vi "Update.vi"(8 "error in (no error)":errorcluster, 10 "Message in":refnum<class "UpdateMessage.lvclass">, 11 "Autofocus in":refnum<class "Autofocus.lvclass">) -> (0 "error out":errorcluster, 3 "Autofocus out":refnum<class "Autofocus.lvclass">)   [LabVIEW 2012, in "Autofocus.lvclass"]
doc: "The update method processes the command 'update'. \n\nThe command 'update' is used for receiving new values to be set to the private data of the class. This could be seen as a public set method for setting new parameters to the private class data."
uses:
  Autofocus.lvclass
  <vilib>/Distrio/Murmex/UpdateMessage/UpdateMessage.lvclass
  Sharpness Measure.ctl
  Autofocus.lvclass/Autofocus.ctl
  image acquisition mode.ctl
  ROI size.ctl
  Search algorithm.ctl
  <vilib>/Distrio/Murmex/Murmex/Murmex.lvclass
panel:
  # "This method is called when the UPDATE\ntrigger is sent. \n\nOverride this method when your component needs to\nrespond to this trigger. \n\nCall parent for proper implementation"
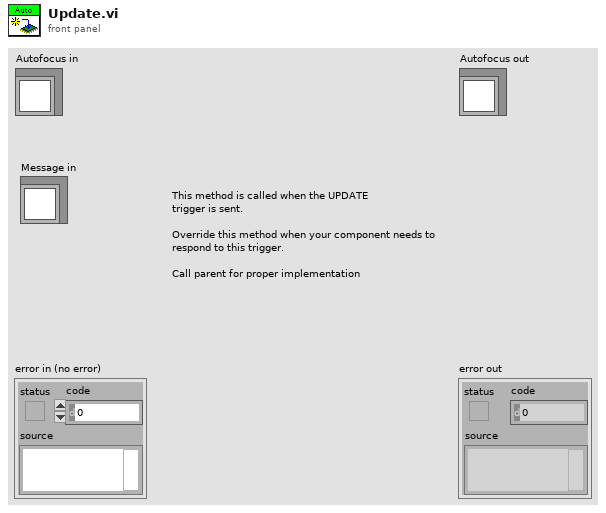
[diagram p1: front panel]
types:
  T1 = typedef "Autofocus.lvclass/Sharpness Measure.ctl" = enum16{"Vol4", "Gradient Square"}
  T2 = typedef "Autofocus.lvclass/image acquisition mode.ctl" = enum16{"Focus Stack", "Single Frame"}
  T3 = typedef "Autofocus.lvclass/Search algorithm.ctl" = enum16{"Hill Climbing", "HC+GS"}
  T4 = typedef "Autofocus.lvclass/ROI size.ctl" = u16
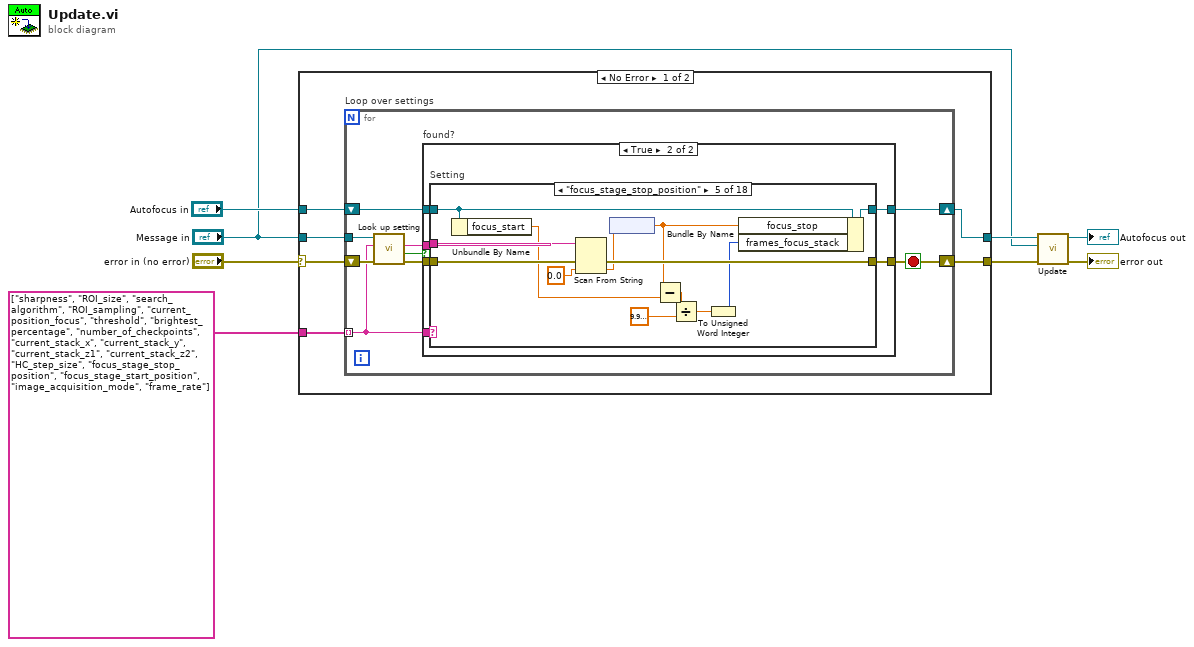
[diagram p0: block diagram]
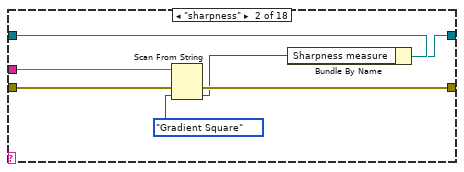
[diagram p4: hidden frame]
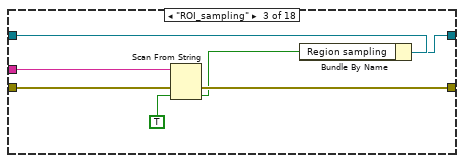
[diagram p5: hidden frame]
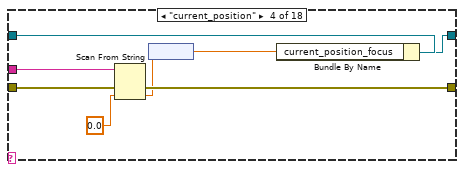
[diagram p6: hidden frame]
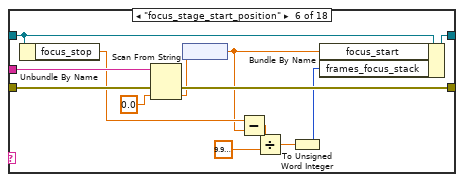
[diagram p7: hidden frame]
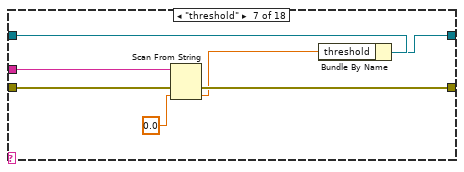
[diagram p8: hidden frame]
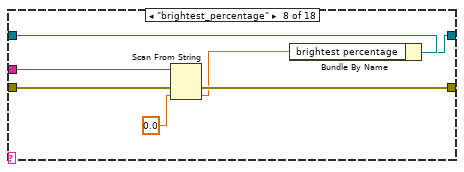
[diagram p9: hidden frame]
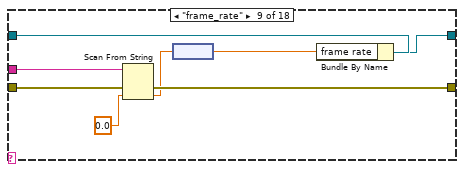
[diagram p10: hidden frame]
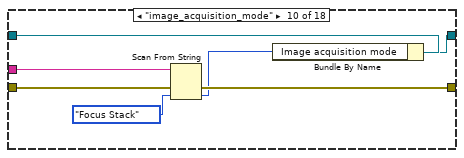
[diagram p11: hidden frame]
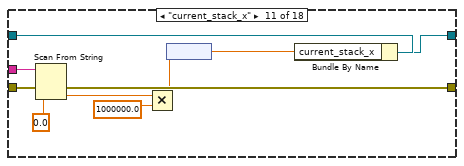
[diagram p12: hidden frame]
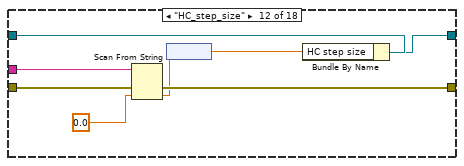
[diagram p13: hidden frame]
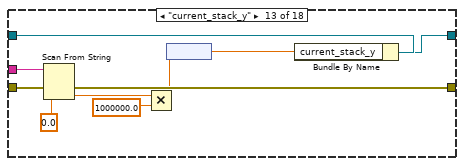
[diagram p14: hidden frame]
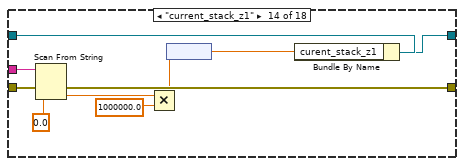
[diagram p15: hidden frame]
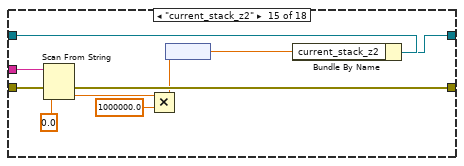
[diagram p16: hidden frame]
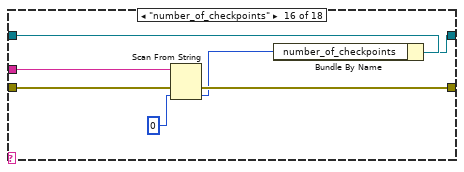
[diagram p17: hidden frame]
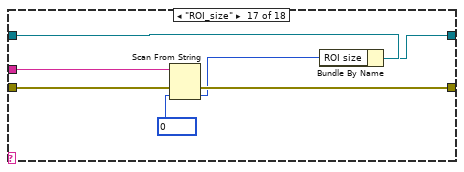
[diagram p18: hidden frame]
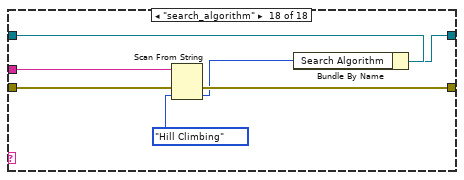
[diagram p19: hidden frame]
diagram:
  n1 = case shown="No Error" "error in (no error)" {
    selector: "error in (no error)" -> [w14 w181]
    tunnel: "Autofocus in" -> [w10 w180]
    tunnel: [w13 w181] -> w5
    tunnel: string[] ["sharpness", "ROI_size", "search_algorithm", "ROI_sampling", "current_position_focus", "threshold", "brightest_percentage", "number_of_checkpoints", "current_stack_x", "current_stack_y", "current_stack_z1", "current_stack_z2", "HC_step_size", "focus_stage_stop_position", "focus_stage_start_position", "image_acquisition_mode", "frame_rate"] -> [w12 _]
    tunnel: "Message in" -> [w11 _]
    tunnel: [w9 w180] -> w3
    frame No Error {
      n2 = for "Loop over settings" {
        shift-right: [w17] -> w13
        shift-left: w14 -> [w23]
        shift-right: [w18] -> w9
        shift-left: w10 -> [w21]
        tunnel: w12 -> [w16] mode=indexing
        tunnel: w11 -> [w15]
        stop <- w17 stop-if-true
        n3 = call <vilib>:"Look up setting.vi"("error in (no error)"=w23, "tag name"=w16, "UpdateMessage in"=w15) -> ("error out"=w19:errorcluster, "found?"=w22:bool, "value"=w20:string)  [unwired: 5 in, 1 out]
        n4 = case "found?" shown="True" w22 {
          tunnel: w21 -> [w25 w29]
          tunnel: w20 -> [_ w30]
          tunnel: w19 -> [w24 w28]
          tunnel: w16 -> [_ w31]
          tunnel: [w25 w27] -> w18
          tunnel: [w24 w26] -> w17
          frame False {
          }
          frame True {
            n5 = case "Setting" shown="\"focus_stage_stop_position\"" w31 {
              tunnel: w30 -> [_ w39 w45 w53 w66 w79 w86 w93 w101 w108 w118 w126 w136 w146 w156 w163 w166 w177]
              tunnel: w29 -> [w33 w38 w43 w52 w57 w76 w85 w92 w100 w107 w117 w125 w135 w145 w155 w162 w169 w175]
              tunnel: w28 -> [w32 w40 w47 w55 w68 w81 w88 w95 w103 w110 w120 w128 w138 w148 w158 w165 w172 w179]
              tunnel: [w33 w37 w42 w51 w65 w78 w84 w91 w99 w106 w116 w124 w134 w144 w154 w161 w167 w174] -> w27
              tunnel: [w32 w36 w46 w54 w67 w80 w87 w94 w102 w109 w119 w127 w137 w147 w157 w164 w171 w178] -> w26
              frame Default {
              }
              frame "sharpness" {
                n6 = Scan From String(input string=w39, error in=w40, default 1=Sharpness_Measure."Gradient Square" ("Sharpness measure")) -> (error out=w36:errorcluster, output 1=w34:T1)  [unwired: 2 in, 2 out]
                n7 = Bundle By Name(cluster=w38, "Sharpness measure"=w34) -> (w37:refnum<class "Autofocus.lvclass">)
              }
              frame "ROI_sampling" {
                n8 = Scan From String(input string=w45, error in=w47, default 1=TRUE) -> (error out=w46:errorcluster, output 1=w41:bool)  [unwired: 2 in, 2 out]
                n9 = Bundle By Name(cluster=w43, "Region sampling"=w41) -> (w42:refnum<class "Autofocus.lvclass">)
              }
              frame "current_position" {
                n10 = Scan From String(input string=w53, error in=w55, default 1=0.0 ("Settings cluster.current_position")) -> (error out=w54:errorcluster, output 1=w49:dbl)  [unwired: 2 in, 2 out]
                n11 = node(w49) -> (w48:dbl[unit])
                n12 = Bundle By Name(cluster=w52, "current_position_focus"=w48) -> (w51:refnum<class "Autofocus.lvclass">)
              }
              frame "focus_stage_stop_position" {
                n13 = Unbundle By Name(w57) -> ("focus_start"=w56:dbl[unit])
                n14 = Scan From String(input string=w66, error in=w68, default 1=0.0 ("Settings cluster.current_position")) -> (error out=w67:errorcluster, output 1=w63:dbl)  [unwired: 2 in, 2 out]
                n15 = node(w63) -> (w58:dbl[unit])
                n16 = Subtract(x=w58, y=w56) -> (x-y=w62:dbl[unit])
                n17 = Divide(x=w62, y=dbl[unit] 9.999999999999999e-06) -> (x/y=w60:dbl)
                n18 = To Unsigned Word Integer(number=w60) -> (unsigned 16bit integer=w59:u16)
                n19 = Bundle By Name(cluster=w57, "focus_stop"=w58, "frames_focus_stack"=w59) -> (w65:refnum<class "Autofocus.lvclass">)
              }
              frame "focus_stage_start_position" {
                n20 = Unbundle By Name(w76) -> ("focus_stop"=w74:dbl[unit])
                n21 = Scan From String(input string=w79, error in=w81, default 1=0.0 ("Settings cluster.current_position")) -> (error out=w80:errorcluster, output 1=w77:dbl)  [unwired: 2 in, 2 out]
                n22 = node(w77) -> (w73:dbl[unit])
                n23 = Subtract(x=w74, y=w73) -> (x-y=w72:dbl[unit])
                n24 = Divide(x=w72, y=dbl[unit] 9.999999999999999e-06) -> (x/y=w70:dbl)
                n25 = To Unsigned Word Integer(number=w70) -> (unsigned 16bit integer=w69:u16)
                n26 = Bundle By Name(cluster=w76, "focus_start"=w73, "frames_focus_stack"=w69) -> (w78:refnum<class "Autofocus.lvclass">)
              }
              frame "threshold" {
                n27 = Scan From String(input string=w86, error in=w88, default 1=0.0 ("Settings cluster.current_position")) -> (error out=w87:errorcluster, output 1=w82:dbl)  [unwired: 2 in, 2 out]
                n28 = Bundle By Name(cluster=w85, "threshold"=w82) -> (w84:refnum<class "Autofocus.lvclass">)
              }
              frame "brightest_percentage" {
                n29 = Scan From String(input string=w93, error in=w95, default 1=0.0 ("Settings cluster.current_position")) -> (error out=w94:errorcluster, output 1=w89:dbl)  [unwired: 2 in, 2 out]
                n30 = Bundle By Name(cluster=w92, "brightest percentage"=w89) -> (w91:refnum<class "Autofocus.lvclass">)
              }
              frame "frame_rate" {
                n31 = Scan From String(input string=w101, error in=w103, default 1=0.0 ("Settings cluster.current_position")) -> (error out=w102:errorcluster, output 1=w97:dbl)  [unwired: 2 in, 2 out]
                n32 = node(w97) -> (w96:dbl[unit])
                n33 = Bundle By Name(cluster=w100, "frame rate"=w96) -> (w99:refnum<class "Autofocus.lvclass">)
              }
              frame "image_acquisition_mode" {
                n34 = Scan From String(input string=w108, error in=w110, default 1=image_acquisition_mode."Focus Stack" ("Settings cluster.Image acquisition mode")) -> (error out=w109:errorcluster, output 1=w105:T2)  [unwired: 2 in, 2 out]
                n35 = Bundle By Name(cluster=w107, "Image acquisition mode"=w105) -> (w106:refnum<class "Autofocus.lvclass">)
              }
              frame "current_stack_x" {
                n36 = Scan From String(input string=w118, error in=w120, default 1=0.0 ("Settings cluster.current_stack_x")) -> (error out=w119:errorcluster, output 1=w112:dbl)  [unwired: 2 in, 2 out]
                n37 = Multiply(x=w112, y=1000000.0) -> (x*y=w111:dbl)
                n38 = node(w111) -> (w114:dbl[unit])
                n39 = Bundle By Name(cluster=w117, "current_stack_x"=w114) -> (w116:refnum<class "Autofocus.lvclass">)
              }
              frame "HC_step_size" {
                n40 = Scan From String(input string=w126, error in=w128, default 1=0.0 ("Settings cluster.current_stack_x")) -> (error out=w127:errorcluster, output 1=w123:dbl)  [unwired: 2 in, 2 out]
                n41 = node(w123) -> (w121:dbl[unit])
                n42 = Bundle By Name(cluster=w125, "HC step size"=w121) -> (w124:refnum<class "Autofocus.lvclass">)
              }
              frame "current_stack_y" {
                n43 = Scan From String(input string=w136, error in=w138, default 1=0.0 ("Settings cluster.current_stack_x")) -> (error out=w137:errorcluster, output 1=w130:dbl)  [unwired: 2 in, 2 out]
                n44 = Multiply(x=w130, y=1000000.0) -> (x*y=w129:dbl)
                n45 = node(w129) -> (w132:dbl[unit])
                n46 = Bundle By Name(cluster=w135, "current_stack_y"=w132) -> (w134:refnum<class "Autofocus.lvclass">)
              }
              frame "current_stack_z1" {
                n47 = Scan From String(input string=w146, error in=w148, default 1=0.0 ("Settings cluster.current_stack_x")) -> (error out=w147:errorcluster, output 1=w140:dbl)  [unwired: 2 in, 2 out]
                n48 = Multiply(x=w140, y=1000000.0) -> (x*y=w139:dbl)
                n49 = node(w139) -> (w142:dbl[unit])
                n50 = Bundle By Name(cluster=w145, "curent_stack_z1"=w142) -> (w144:refnum<class "Autofocus.lvclass">)
              }
              frame "current_stack_z2" {
                n51 = Scan From String(input string=w156, error in=w158, default 1=0.0 ("Settings cluster.current_stack_x")) -> (error out=w157:errorcluster, output 1=w151:dbl)  [unwired: 2 in, 2 out]
                n52 = Multiply(x=w151, y=1000000.0) -> (x*y=w150:dbl)
                n53 = node(w150) -> (w152:dbl[unit])
                n54 = Bundle By Name(cluster=w155, "current_stack_z2"=w152) -> (w154:refnum<class "Autofocus.lvclass">)
              }
              frame "number_of_checkpoints" {
                n55 = Scan From String(input string=w163, error in=w165, default 1=u16 0 ("Settings cluster.current_position")) -> (error out=w164:errorcluster, output 1=w159:u16)  [unwired: 2 in, 2 out]
                n56 = Bundle By Name(cluster=w162, "number_of_checkpoints"=w159) -> (w161:refnum<class "Autofocus.lvclass">)
              }
              frame "ROI_size" {
                w170 = T4 0 items=["50x50"=50, "100x100"=100, "250x250"=250] ("ROI size")
                n57 = Scan From String(input string=w166, error in=w172, default 1=w170) -> (error out=w171:errorcluster, output 1=w168:T4)  [unwired: 2 in, 2 out]
                n58 = Bundle By Name(cluster=w169, "ROI size"=w168) -> (w167:refnum<class "Autofocus.lvclass">)
              }
              frame "search_algorithm" {
                n59 = Scan From String(input string=w177, error in=w179, default 1=Search_algorithm."Hill Climbing" ("Search Algorithm")) -> (error out=w178:errorcluster, output 1=w173:T3)  [unwired: 2 in, 2 out]
                n60 = Bundle By Name(cluster=w175, "Search Algorithm"=w173) -> (w174:refnum<class "Autofocus.lvclass">)
              }
            }
          }
        }
      }
    }
    frame Error {
    }
  }
  n61 = call-parent "Update.vi"("error in (no error)"=w5, "Message in"="Message in", "Murmex in"=w3) -> ("error out"=→"error out":errorcluster, "Murmex out"=→"Autofocus out":refnum<class "Autofocus.lvclass">)  [unwired: 7 in]
